vi "Bitpacking test.vi"() -> ()   [LabVIEW 2019]
uses:
  <instrlib>/_niInstr/DSP/v1/Shared/Public/IQ Data.ctl
  <instrlib>/FlexRIO/DRAM FIFO/v2/FPGA/DRAM FIFO/FIFO Depth.ctl
  <vilib>/Platform/TimedLoop/XDataNode/timing_clust.ctl
  <vilib>/Platform/TimedLoop/XDataNode/nitl_modes.ctl
  <vilib>/Platform/TimedLoop/XDataNode/wakeup.ctl
  <instrlib>/FlexRIO/DRAM FIFO/v2/FPGA/DRAM FIFO/Private/DRAM FIFO U512/Create 512x1 DRAM FIFO.vi
  <vilib>/rvi/DataTransferAndStorage/Container/Common/niFpgaContainerGetUniqueNameForEmu.vi
  <vilib>/rvi/DataTransferAndStorage/Container/Common/niFpgaContainerSetEmuInfo.vi
  <vilib>/rvi/eio/common/nirviEmuReportErrorAndStop.vi
  <vilib>/rvi/Emulation/niFpgaSctlEmulationGetInTimedLoop.vi
  <vilib>/rvi/Emulation/niFpgaEmulationReportErrorSimple.vi
  <vilib>/rvi/Emulation/niFpgaGetClockAttributes.vi
  <vilib>/rvi/Emulation/niFpgaCriticalErrorInLSC.vi
  <instrlib>/_niInstr/Data Formatting/v1/FPGA/Private/Convert/U64 array to Boolean Array.vi
  <instrlib>/_niInstr/Basic Elements/v1/FPGA/Private/Count Up U32.vi
  <instrlib>/_niInstr/Data Formatting/v1/FPGA/Private/Convert/FXP(+-,12,1) array to Boolean Array.vi
  <instrlib>/_niInstr/Data Formatting/v1/FPGA/Private/Convert/Boolean Array to FXP(+-,12,1) Array.vi
  <vilib>/rvi/DataTransferAndStorage/Container/Common/niFpgaContainerExecOnDevCompGetState.vi
  <vilib>/rvi/Emulation/niFpgaEmulationIsFPGAContextNoSignature.vi
  <vilib>/rvi/errors/niFpgaSetErrorForExecOnDevCompSimple.vi
  <vilib>/rvi/FIFO/Fifo_Resource/nirvififoEmulationSetSize.vi
  <vilib>/rvi/FIFO/Fifo_Resource/nirviFifoEmulationQueueMgr.vi
  <instcachedir>/0/nirviFifoEmulationQueueMgr_E5CAEC123FF24DC58D834DCA3CDAA9B5.lvgen/nirviFifoEmulationQueueMgr_E5CAEC123FF24DC58D834DCA3CDAA9B5_011.vi
  <vilib>/rvi/FIFO/Fifo_Resource/nirvififoEmulationDetermineInputValidOut.vi
  <vilib>/rvi/FIFO/Fifo_Resource/nirvififoEmulationCreateLock.vi
  <vilib>/rvi/Emulation/niFpgaProcessEmulError.vi
  <vilib>/rvi/FIFO/Fifo_Resource/nirvififoEmulationObtainLock.vi
  <vilib>/rvi/FIFO/Fifo_Resource/nirvififoEmulationReleaseLock.vi
  <vilib>/rvi/occurrence/nirviWaitOnOccurrenceBase.vi
  <vilib>/rvi/errors/nirviReportUnexpectedCaseInternalError.vi
  <vilib>/rvi/errors/nirviReportUnexpectedCaseInternalError (U32).vi
  <vilib>/Utility/error.llb/Clear Errors.vi
  <vilib>/rvi/interface/RandomDataEmulation/niFpgaRandomDataHandleErrors.vi
  <instrlib>/FlexRIO/DRAM FIFO/v2/FPGA/DRAM FIFO/Pack Boolean Array.vi
  <vilib>/Platform/TimedLoop/XDataNode/XDataNode.xnode
  <vilib>/rvi/LocalResourceManager/LocalResourceManager.xnode
  <vilib>/rvi/DataTransferAndStorage/Container/XNode/niFpgaContainer.xnode
  <vilib>/rvi/FIFO/Fifo_Resource/niFpgaFifoEmulationRefIn.vi
  <vilib>/Platform/TimedLoop/XDataNode/XDNodeRunTimeDep.lvlib
  <instrlib>/FlexRIO/DRAM FIFO/v2/FPGA/DRAM FIFO/DRAM FIFO v2 FPGA.lvclass
  <instrlib>/_niInstr/Data Formatting/v1/FPGA/niInstr Data Formatting v1 FPGA.lvlib
  <instrlib>/_niInstr/Basic Elements/v1/FPGA/niInstr Basic Elements v1 FPGA.lvlib
  <instrlib>/FlexRIO/DRAM FIFO/v2/FPGA/DRAM FIFO/Private/DRAM FIFO U512/DRAM FIFO U512 v2 FPGA.lvclass
  SubVIs/Utility/FPGA Utility.lvlib
  <instrlib>/_niInstr/DSP/v1/Shared/niInstr DSP v1 Shared.lvlib
panel:
  in  "tone data":T1[](array[typedef])=[{"I"=0.01000213623046875, "Q"=0.0, "overflow"=FALSE}, {"I"=0.01999664306640625, "Q"=0.0, "overflow"=FALSE}, {"I"=0.029998779296875, "Q"=0.0, "overflow"=FALSE}, {"I"=0.04000091552734375, "Q"=0.0, "overflow"=FALSE}, {"I"=0.0500030517578125, "Q"=0.0, "overflow"=FALSE}, {"I"=0.05999755859375, "Q"=0.0, "overflow"=FALSE}, {"I"=0.06999969482421875, "Q"=0.0, "overflow"=FALSE}, {"I"=0.0800018310546875, "Q"=0.0, "overflow"=FALSE}, {"I"=0.089996337890625, "Q"=0.0, "overflow"=FALSE}, {"I"=0.09999847412109375, "Q"=0.0, "overflow"=FALSE}, {"I"=0.1100006103515625, "Q"=0.0, "overflow"=FALSE}, {"I"=0.12000274658203125, "Q"=0.0, "overflow"=FALSE}, {"I"=0.12999725341796875, "Q"=0.0, "overflow"=FALSE}, {"I"=0.1399993896484375, "Q"=0.0, "overflow"=FALSE}, {"I"=0.15000152587890625, "Q"=0.0, "overflow"=FALSE}, {"I"=0.160003662109375, "Q"=0.0, "overflow"=FALSE}]
  out "data out 2":fxp<+/-,12,1>[](array[numeric])
  out "data out":fxp<+/-,12,1>[](array[numeric])
  out "Number of Elements to Read":u32
  in  "reset":bool
  in  "flush data":bool
  out "count in":u32
  out "count out":u32
  out "count pack":u32
  in  "input valid":bool
  out "out data valid":bool
  in  "in data u64":u64[](array[numeric]) format="%016x"
  out "elements per valid output":i32
  out "packed data valid":bool
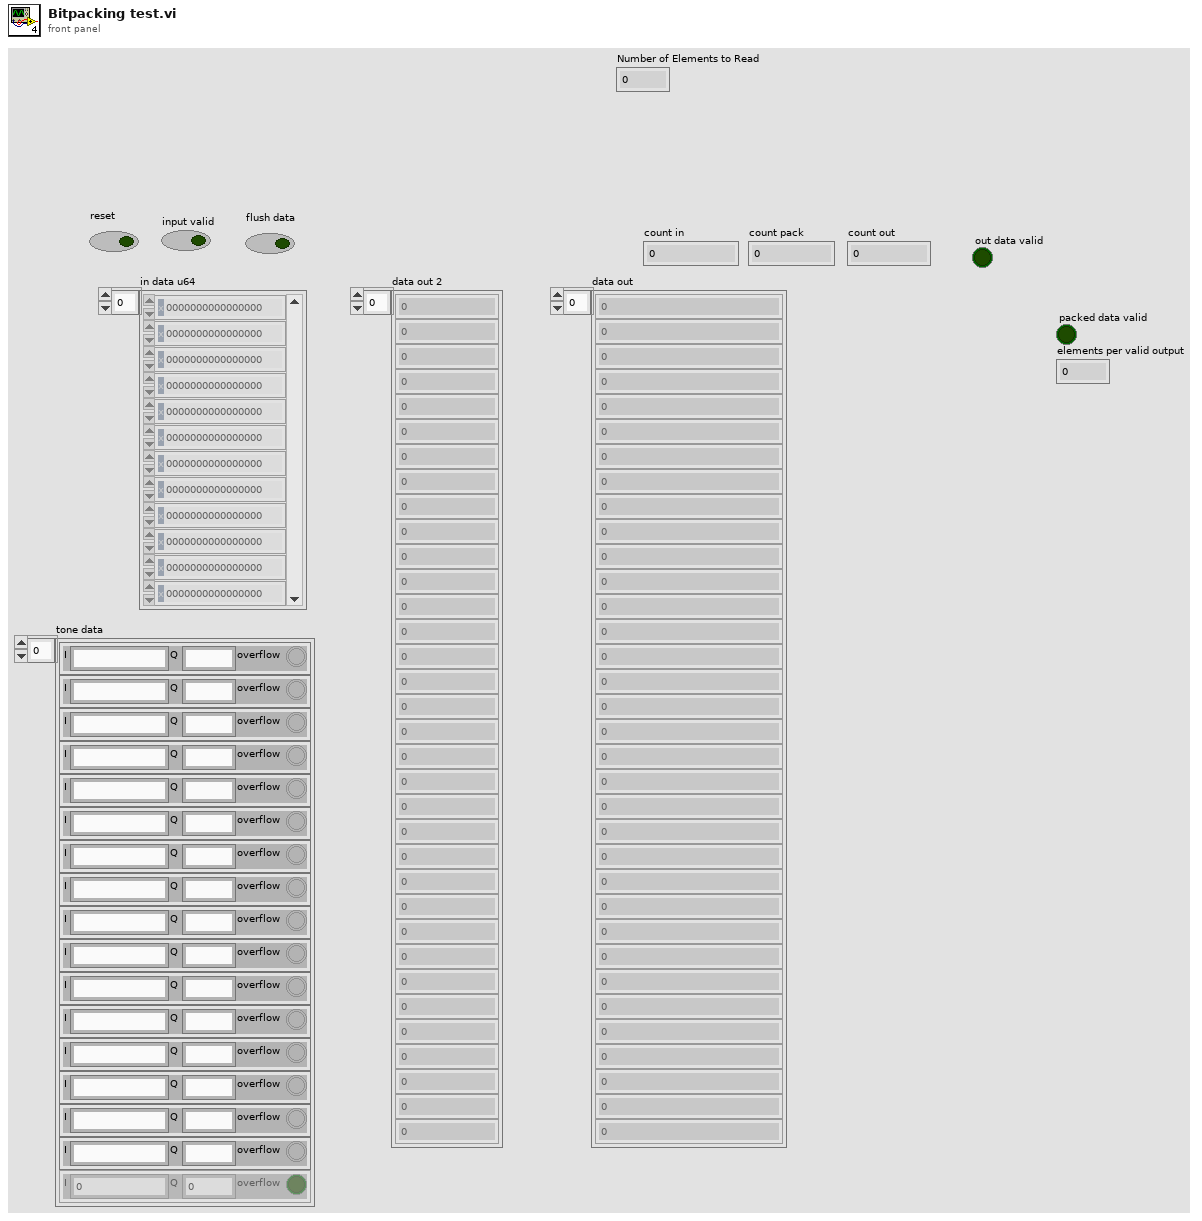
[diagram p1: front panel]
types:
  T1 = typedef "niInstr DSP v1 Shared.lvlib/IQ Data.ctl" = cluster{"I":fxp<+/-,18,1>, "Q":fxp<+/-,18,1>, "overflow":bool}
  T2 = typedef "DRAM FIFO v2 FPGA.lvclass/FIFO Depth.ctl" = u8
  T3 = typedef "XDNodeRunTimeDep.lvlib/timing_clust.ctl" = cluster{"Expected End [f-1]":u64, "Actual End [f-1]":u64, "Finished Late? [f-1]":bool, "Expected End [i-1]":u64, "Actual End [i-1]":u64, "Finished Late? [i-1]":bool, "Expected Start [i]":u64, "Actual Start [i]":u64, "Expected Start [f]":u64, "Actual Start [f]":u64, "Source Name":string, "Structure Name":string, "Period":i64, "Deadline":i64, "Offset":i64, "Start":i64, "Priority":i32, "Timeout":i32, "Mode":T4, "Wakeup Reason":T5, "Error":errorcluster, "Source Type":string, "Secondary Source Type":string, "Global End Time":u64, "Global Start Time":u64, "Frame Duration":u64, "Iteration Duration":u64, "Assigned CPU":i32, "I/O Scan Engine Mode":u32}
  T4 = typedef "XDNodeRunTimeDep.lvlib/nitl_modes.ctl" = enum32{"No Change", "Process missed periods, maintain original phase", "Discard missed periods, maintain original phase", "Process missed periods, ignore original phase", "Discard missed periods, ignore original phase"}
  T5 = typedef "XDNodeRunTimeDep.lvlib/wakeup.ctl" = enum32{"Normal", "Aborted", "Asynchronous wakeup", "Timing source error", "Timed loop error", "Timeout"}
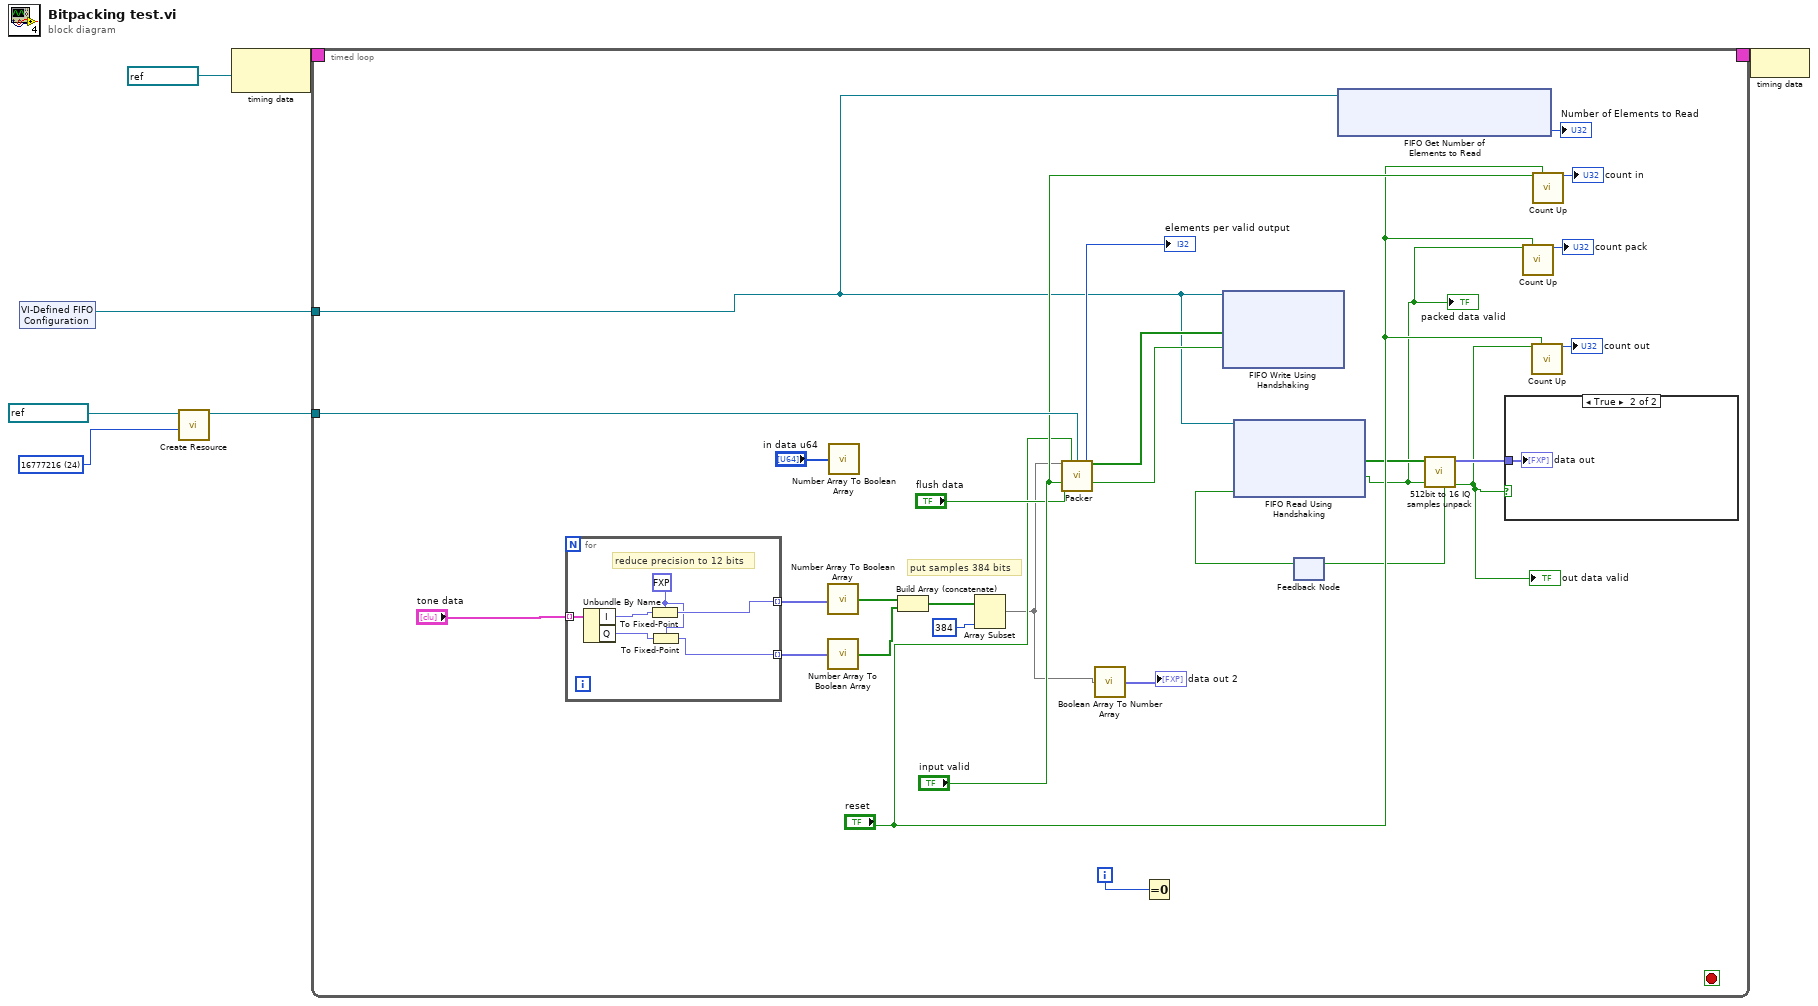
[diagram p0: block diagram]
diagram:
  w4 = T2 24 items=["4"=2, "8"=3, "16"=4, "32"=5, "64"=6, "128"=7, "256"=8, "512"=9, "1024"=10, "2048"=11, "4096"=12, "8192"=13, "16384"=14, "32768"=15, "65536"=16, "131072"=17, "262144"=18, "524288"=19, "1048576"=20, "2097152"=21, "4194304"=22, "8388608"=23, "16777216"=24, "33554432"=25, "67108864"=26, "134217728"=27, "268435456"=28, "536870912"=29, "1073741824"=30, "2147483648"=31, "4294967296"=32] ("actual # of DRAM elements")
  n1 = xnode "VI-Defined FIFO Configuration"() -> ("FIFO Out"=w1:refnum<k21>)
  n2 = call-poly <instrlib>:"Create Resource.vi"("actual # of DRAM elements"=w4, "memory refnum"=refnum<k21> "RX memo") -> ("DRAM FIFO ref out"=w3:refnum<class "DRAM FIFO v2 FPGA.lvclass">)  [unwired: 9 in]
  n3 = node-c288(refnum<k21> "195MHz" ("Source Name")) -> (w7:T3)
  n4 = timed-loop {
    timing: w7 -> [_]
    timing-out: [_] -> w6
    tunnel: w3 -> [w36]
    tunnel: w1 -> [w17]
    i -> [w27]
    stop <- _ stop-if-true
    # "put samples 384 bits"
    n5 = for {
      tunnel: [w41] -> w35 mode=indexing
      tunnel: [w38] -> w31 mode=indexing
      tunnel: "tone data" -> [w43] mode=indexing
      w40 = fxp<+/-,12,1> 0.0 ("fixed-point type")
      # "reduce precision to 12 bits"
      n6 = Unbundle By Name(w43) -> ("I"=w42:fxp<+/-,18,1>, "Q"=w39:fxp<+/-,18,1>)
      n7 = To Fixed-Point(fixed-point type=w40, number=w42) -> (fixed-point=w41:fxp<+/-,12,1>)
      n8 = To Fixed-Point(fixed-point type=w40, number=w39) -> (fixed-point=w38:fxp<+/-,12,1>)
    }
    n9 = call-poly <instrlib>:"Number Array To Boolean Array.vi"("data in"=w35) -> ("data out"=w34:bool[])  [unwired: 14 in]
    n10 = call-poly <instrlib>:"Number Array To Boolean Array.vi"("data in"=w31) -> ("data out"=w30:bool[])  [unwired: 14 in]
    n11 = call-poly <instrlib>:"Number Array To Boolean Array.vi"("data in"="in data u64") -> ()  [unwired: 14 in, 1 out]
    n12 = Build Array (concatenate)(w34, w30) -> (w32:bool[])
    n13 = Array Subset(array=w32, length=384) -> (w8:bool[])  [unwired: 1 in]
    n14 = call-poly <instrlib>:"Packer.vi"("data in"=w8, "reset"="reset", "DRAM FIFO in"=w36, "flush data"="flush data", "input valid"="input valid") -> ("elements per valid output"=→"elements per valid output":i32, "data out"=w19:bool[], "output valid"=w18:bool)  [unwired: 8 in]
    n15 = call-poly <instrlib>:"Boolean Array To Number Array.vi"("data in"=w8) -> ("data out"=→"data out 2":fxp<+/-,12,1>[])  [unwired: 14 in]
    n16 = Equal To 0?(x=w27) -> ()  [unwired: 1 out]
    n17 = xnode "FIFO Write Using Handshaking"("Element"=w19, "Input Valid"=w18, "FIFO In"=w17) -> ()  [unwired: 2 out]
    n18 = feedback #1() -> (w12:bool)  [unwired: 1 in]
    n19 = xnode "FIFO Read Using Handshaking"("Ready for Output"=w12, "FIFO In"=w17) -> ("Element"=w15:bool[], "Output Valid"=w14:bool)  [unwired: 1 out]
    "packed data valid" <- w14
    n20 = xnode "FIFO Get Number of Elements to Read"("FIFO In"=w17) -> ("Number of Elements to Read"=→"Number of Elements to Read":u32)  [unwired: 1 out]
    n21 = call "512bit to 16 IQ samples unpack.vi"("input valid"=w14, "data in"=w15) -> ("output valid"=w10:bool, "data out"=w11:fxp<+/-,12,1>[], "ready for input"=w13:bool)  [unwired: 7 in]
    "out data valid" <- w10
    n22 = feedback-in #1(w13) -> ()
    n23 = case shown="True" w10 {
      tunnel: w11 -> [_ w37]
      frame False {
      }
      frame True {
        "data out" <- w37
      }
    }
    n24 = call-poly <instrlib>:"Count Up.vi"("increment"=w14, "reset"="reset") -> ("count out"=→"count pack":u32)  [unwired: 13 in]
    n25 = call-poly <instrlib>:"Count Up.vi"("increment"=w10, "reset"="reset") -> ("count out"=→"count out":u32)  [unwired: 13 in]
    n26 = call-poly <instrlib>:"Count Up.vi"("increment"="input valid", "reset"="reset") -> ("count out"=→"count in":u32)  [unwired: 13 in]
  }
  n27 = node-c288(w6) -> ()
